vi "Create Sensor Channel.vi"(5 "regular expression":string="[.]", 6 "Channel":T2, 7 "Object":i32=1, 8 "error in (no error)":errorcluster, 9 "RDB Signalname":string, 10 "RDB Receive Objects":string, 11 "Item Ref in":T1 format="%.0x") -> (0 "error out":errorcluster, 3 "pkid":u32)   [LabVIEW 2018, in "Vires VTD System Explorer.lvlib"]
uses:
  Vires VTD System Explorer.lvlib
  <vilib>/NI Veristand/Custom Device API/Custom Device Channel.ctl
  <vilib>/NI Veristand/Custom Device API/Custom Device Channel Type.ctl
  <vilib>/NI Veristand/Custom Device API/Custom Device Item Ref.ctl
  <vilib>/xnet/xnet.llb/XNET String To IO Name (Signal).vi
  Shared/Constants.vi
  <vilib>/NI Veristand/Custom Device API/Custom Device API.lvlib
  Shared/Vires VTD Shared.lvlib
  <resource>/objmgr/xnet.rc
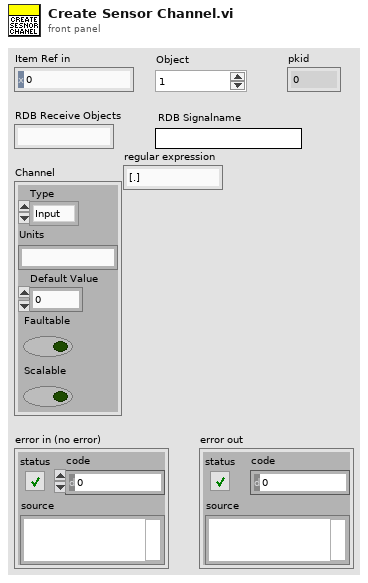
[diagram p1: front panel]
types:
  T1 = typedef "Custom Device API.lvlib/Custom Device Item Ref.ctl" = u64
  T2 = typedef "Custom Device API.lvlib/Custom Device Channel.ctl" = cluster{"Type":T3, "Units":string, "Default Value":dbl, "Faultable":bool, "Scalable":bool}
  T3 = typedef "Custom Device API.lvlib/Custom Device Channel Type.ctl" = enum16{"Input", "Output"}
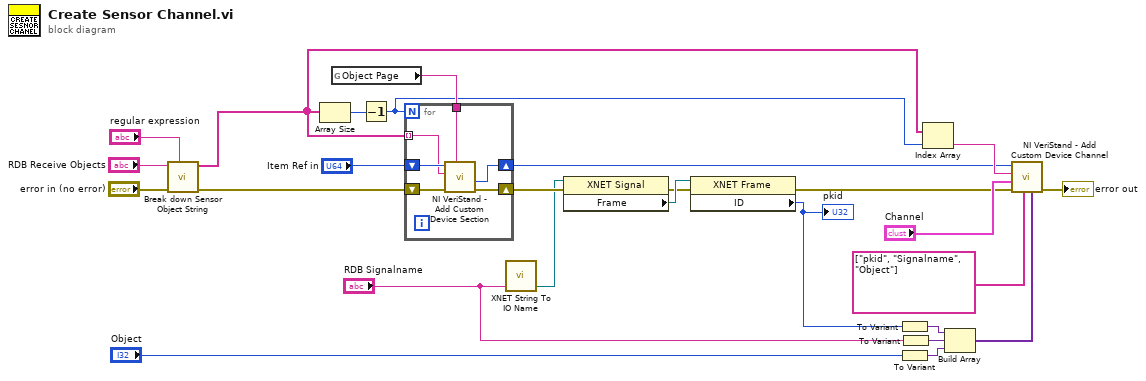
[diagram p0: block diagram]
diagram:
  n1 = call "Break down Sensor Object String.vi"("regular expression"="regular expression", "Error in"="error in (no error)", "Input String"="RDB Receive Objects") -> ("Error Out"=w21:errorcluster, "Output"=w19:string[])  [unwired: 7 in]
  n2 = Array Size(array=w19) -> (size(s)=w20:i32)
  n3 = global read "Constants.vi" "Object Page"() -> (w23:string)
  n4 = Decrement(x=w20) -> (x-1=w18:i32)
  n5 = for {
    N: w18 -> [_]
    tunnel: w23 -> [w31]
    shift-right: [w27] -> w16
    shift-left: "Item Ref in" -> [w32]
    shift-right: [w29] -> w7
    shift-left: w21 -> [w30]
    tunnel: w19 -> [w28] mode=indexing
    n6 = call <vilib>:"NI VeriStand - Add Custom Device Section.vi"("GUID (Default Section)"=w31, "error in (no error)"=w30, "Section Name"=w28, "Parent Ref in"=w32) -> ("error out"=w29:errorcluster, "Section Ptr"=w27:T1)  [unwired: 4 in, 2 out]
  }
  n7 = call-poly <vilib>:"XNET String To IO Name.vi"("string"="RDB Signalname") -> ("XNET Signal"=w5:refnum<k21>)  [unwired: 4 out]
  n8 = property class="XNET Signal"(reference=w5, error in=w7) -> (error out=w8:errorcluster, "Frame"=w9:refnum<k21>)  [unwired: 1 out]
  n9 = property class="XNET Frame"(reference=w9, error in=w8) -> (error out=w6:errorcluster, "ID"=w2:u32)  [unwired: 1 out]
  "pkid" <- w2
  n10 = To Variant(anything=w2) -> (Variant=w3:variant)
  n11 = To Variant(anything="Object") -> (Variant=w11:variant)
  n12 = To Variant(anything="RDB Signalname") -> (Variant=w14:variant)
  n13 = Index Array(array=w19, index=w18) -> (element=w17:string)
  n14 = Build Array(w3, w14, w11) -> (w13:variant[])
  n15 = call <vilib>:"NI VeriStand - Add Custom Device Channel.vi"("Property Values"=w13, "Property names"=string[] ["pkid", "Signalname", "Object"], "error in (no error)"=w6, "Channel"="Channel", "Channel Name"=w17, "Parent Ref in"=w16) -> ("error out"=→"error out":errorcluster)  [unwired: 2 in, 3 out]
